vi "UMLEditor_FindObject.vi"(6 "FindManyEdges(False)":bool, 7 "offset":T1 {"y" format="%.2f"; "x" format="%.2f"}, 8 "error in":errorcluster, 9 "IgnoreTheseNodes":refnum<class "AbstractNode.lvclass">[](array[class]), 10 "graphics":refnum<class "Graphics.lvclass">, 11 "graph":refnum<class "Graph.lvclass">) -> (0 "error out":errorcluster, 1 "NodeFound":bool, 2 "node":refnum<class "AbstractNode.lvclass">, 3 "edge":refnum<class "AbstractEdge.lvclass">, 4 "Edges":refnum<class "AbstractEdge.lvclass">[](array[class]), 5 "EdgeFound":bool)   [LabVIEW 2012]
uses:
  <resource>/Framework/Providers/Open_GDS/UML/Graphics_class/Graphics.lvclass
  <resource>/Framework/Providers/Open_GDS/UML/AbstractEdge_class/AbstractEdge.lvclass
  <resource>/Framework/Providers/Open_GDS/UML/Graph_class/Graph.lvclass
  <resource>/Framework/Providers/Open_GDS/UML/AbstractNode_class/AbstractNode.lvclass
  <resource>/Framework/Providers/Open_GDS/UML/General/Point/Point Point2D.ctl
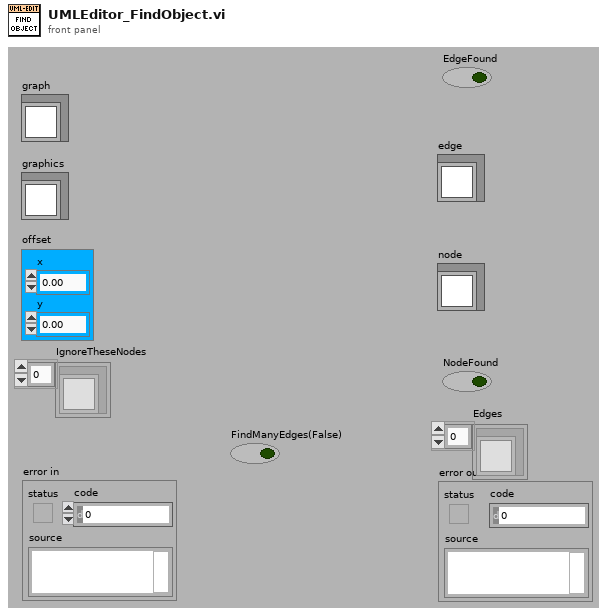
[diagram p1: front panel]
types:
  T1 = typedef "Point Point2D.ctl" = cluster{"x":dbl, "y":dbl}
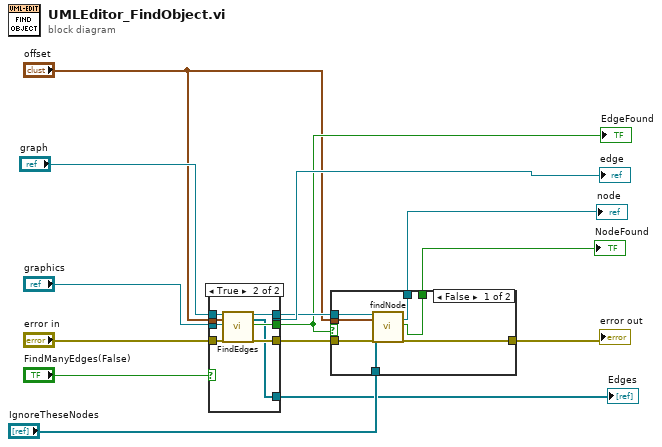
[diagram p0: block diagram]
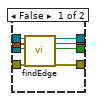
[diagram p2: hidden frame]
diagram:
  n1 = case shown="True" "FindManyEdges(False)" {
    tunnel: "graphics" -> [w22 w28]
    tunnel: [w21 _] -> w13
    tunnel: "offset" -> [w20 w29]
    tunnel: "graph" -> [w19 w30]
    tunnel: [w18 w24] -> w8
    tunnel: "error in" -> [w17 w27]
    tunnel: [w16 w26] -> w6
    tunnel: [w15 w25] -> w4
    tunnel: [_ w23] -> w1
    frame False {
      n2 = call-dynamic "findEdge.vi"("reference"=w19, "point2D"=w20, "GraphicsRef"=w22, "error in (no error)"=w17) -> ("reference out"=w18:refnum<class "Graph.lvclass">, "edge"=w21:refnum<class "AbstractEdge.lvclass">, "found"=w15:bool, "error out"=w16:errorcluster)  [unwired: 12 in]
    }
    frame True {
      n3 = call-dynamic "FindEdges.vi"("reference"=w30, "point2D"=w29, "GraphicsRef"=w28, "error in (no error)"=w27) -> ("reference out"=w24:refnum<class "Graph.lvclass">, "Edges"=w23:refnum<class "AbstractEdge.lvclass">[], "found"=w25:bool, "error out"=w26:errorcluster)  [unwired: 12 in]
    }
  }
  "edge" <- w13
  "EdgeFound" <- w4
  "Edges" <- w1
  n4 = case shown="False" w4 {
    tunnel: [w37 _] -> w12
    tunnel: [w36 _] -> w11
    tunnel: "offset" -> [w35 _]
    tunnel: "IgnoreTheseNodes" -> [w34 _]
    tunnel: w8 -> [w33 _]
    tunnel: w6 -> [w32 w38]
    tunnel: [w31 w38] -> w5
    frame False {
      n5 = call-dynamic "findNode.vi"("reference"=w33, "point2D"=w35, "IgnoreTheseNodes"=w34, "error in (no error)"=w32) -> ("node"=w37:refnum<class "AbstractNode.lvclass">, "found"=w36:bool, "error out"=w31:errorcluster)  [unwired: 12 in, 1 out]
    }
    frame True {
    }
  }
  "node" <- w12
  "error out" <- w5
  "NodeFound" <- w11
